vi "DSF.Engine.Transfer Group.Set Transfers.vi"(10 "Transfers":refnum<class "DSF.Engine.Transfer.lvclass">[](array[class]), 11 "Transfer Group in":refnum<class "DSF.Engine.Transfer Group.lvclass">) -> (3 "Transfer Group out":refnum<class "DSF.Engine.Transfer Group.lvclass">)   [LabVIEW 2017, in "DSF.Engine.lvlib" / "DSF.Engine.Transfer Group.lvclass"]
uses:
  DSF.Engine.Transfer Group.lvclass
  DSF.Engine.Transfer.lvclass
  DSF.Engine.Transfer Group.lvclass/DSF.Engine.Transfer Group.ctl
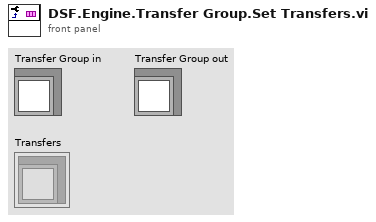
[diagram p1: front panel]
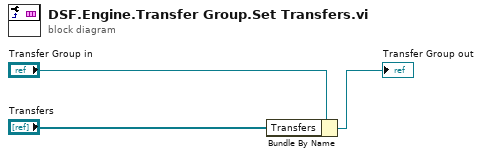
[diagram p0: block diagram]
diagram:
  n1 = Bundle By Name(cluster="Transfer Group in", "Transfers"="Transfers") -> (→"Transfer Group out":refnum<class "DSF.Engine.Transfer Group.lvclass">)
